vi "RingdownData.vi"(7 "LVWSR":refnum<class "Web Request.lvclass">, 11 "Write?":u8) -> ()   [LabVIEW 2014]
uses:
  <vilib>/wsapi/Web Request.lvclass
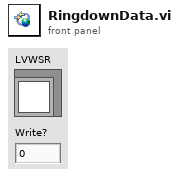
[diagram p1: front panel]
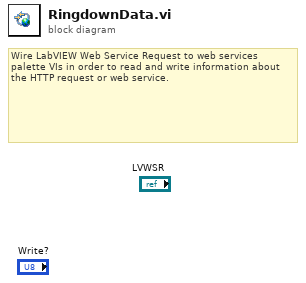
[diagram p0: block diagram]
diagram:
  # "Wire LabVIEW Web Service Request to web services palette VIs in order to read and write information about the HTTP request or web service."
